vi "FTW-CodeGen-GetHelp.vi"(0 "State In":T4 {"Cache"."TotalCodeGens" format="CodeGens:   %04d"; "Cache"."TotalAdaptToInputs" format="AdaptTerms: %04d"; "Cache"."FinishedCodegen" format="%_3psec"; "Cache"."ElapsedTilCodegen" format="%_3psec"; "Cache"."AdaptToInputsBegin" format="%.3fmsec\n%<%D:%H:%M:%S%3u>t"}, 5 "XRef":refnum<vi>, 7 "Point":cluster{"Horizontal":i32, "Vertical":i32}) -> (4 "Standard Help Info":T3, 6 "Detailed Help Info":T2, 8 "Subitem Help Info":T1, 10 "Use Detailed Help?":bool, 15 "Use Subitem Help?":bool)   [LabVIEW 2015, in "FTW-SQLite-Insert.xnode"]
uses:
  FTW-CodeGen-State.ctl
  FTW-CodeGen-XNodeCommonState.ctl
  FTW-CodeGen-XNodeAdaptiveTerminal.ctl
  FTW-CodeGen-XNodeAdaptiveTerminal-Controller.ctl
  src/reflection/FTW-Reflection-Types.ctl
  FTW-CodeGen-XNodeAdaptiveTerminalWiringBehavior.ctl
  FTW-SQLite-Insert.xnode
panel:
  # "Inputs"
  # "Outputs"
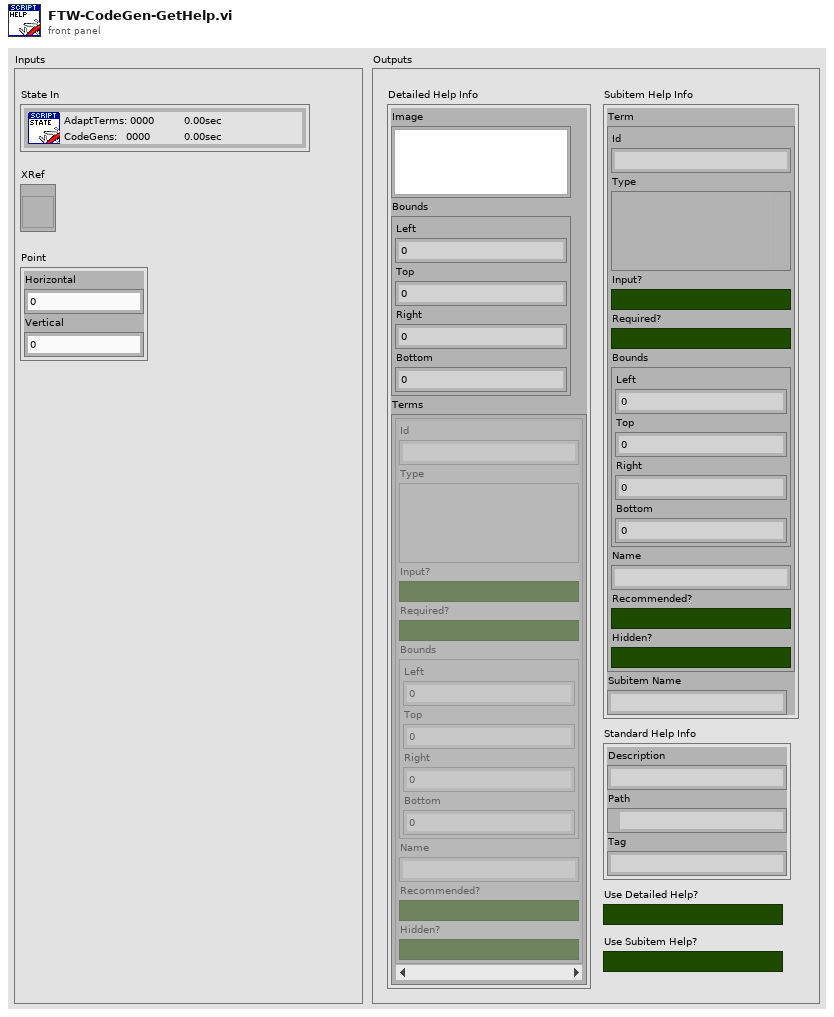
[diagram p1: front panel]
types:
  T1 = cluster{"Term":cluster{"Id":string, "Type":variant, "Input?":bool, "Required?":bool, "Bounds":cluster{"Left":i32, "Top":i32, "Right":i32, "Bottom":i32}, "Name":string, "Recommended?":bool, "Hidden?":bool}, "Subitem Name":string}
  T2 = cluster{"Image":picture, "Bounds":cluster{"Left":i32, "Top":i32, "Right":i32, "Bottom":i32}, "Terms":cluster{"Id":string, "Type":variant, "Input?":bool, "Required?":bool, "Bounds":cluster{"Left":i32, "Top":i32, "Right":i32, "Bottom":i32}, "Name":string, "Recommended?":bool, "Hidden?":bool}[]}
  T3 = cluster{"Description":string, "Path":path, "Tag":string}
  T4 = typedef "FTW-SQLite-Insert.xnode/FTW-CodeGen-State.ctl" = cluster{"Cache":T5}
  T5 = typedef "FTW-CodeGen-XNodeCommonState.ctl" = cluster{"Terms":cluster{"Name":string, "Id":string, "Type":variant, "Bounds":cluster{"Left":i32, "Top":i32, "Right":i32, "Bottom":i32}, "Input?":bool, "Required?":bool, "Recommended?":bool, "Adaptive?":bool, "Hidden?":bool, "Direction":enum32{"Auto", "Up", "Down", "Left", "Right", "Center"}, "Break Wire?":bool, "English Name":string}[], "AdaptiveTerms":T6[], "AdaptiveTerminalsOK":bool, "ForceCodeRegeneration?":bool, "LastGeneration":timestamp, "CodeGenError":errorcluster, "AdaptToInputsBegin":dbl, "ElapsedTilCodegen":dbl, "FinishedCodegen":dbl, "TotalAdaptToInputs":i32, "TotalCodeGens":i32}
  T6 = typedef "FTW-CodeGen-XNodeAdaptiveTerminal.ctl" = cluster{"Config":T7, "ID":string, "ParentIndex":i32, "Wired?":bool, "WiredTypeAllowed?":bool, "LastValidWireName":string, "LastValidWireType":T8, "Followers":i32[]}
  T7 = typedef "FTW-CodeGen-XNodeAdaptiveTerminal-Controller.ctl" = cluster{"AllowedTypes":T8[], "UnconstrainedTypeBehavior":T9, "DefaultType":variant}
  T8 = typedef "FTW-Reflection-Types.ctl" = enum16{"Unknown", "Void", "Array", "Cluster", "LVObject", "Boolean", "I8", "I16", "I32", "I64", "U8", "U16", "U32", "U64", "SGL", "DBL", "EXT", "CSG", "CDB", "CXT", "FXP", "EnumU8", "EnumU16", "EnumU32", "EnumU64", "SGLwithUnit", "DBLwithUnit", "EXTwithUnit", "CSGwithUnit", "CDBwithUnit", "CXTwithUnit", "String", "Path", "Picture", "Tag", "LVVariant", "Timestamp", "WaveformI8", "WaveformI16", "WaveformI32", "WaveformI64", "WaveformU8", "WaveformU16", "WaveformU32", "WaveformU64", "WaveformSGL", "WaveformDBL", "WaveformEXT", "WaveformCSG", "WaveformCDB", "WaveformCXT", "WaveformDigital", "WaveformUnknownType", "DigitalData", "DynamicData", "ExternalData", "FileByteStream", "TDMStream", "dotNET", "ActiveX", "VIServerReference", "VIReference", "ApplicationInstance", "Menu", "ConnectionDataSocket", "ConnectionVISA", "ConnectionBluetooth", "ConnectionIrDA", "ConnectionTCP", "ConnectionUDP", "ConnectionHTTPClient", "ConnectionFTP", "Occurrence", "Notifier", "Queue", "Rendezvous", "Semaphore", "RTFIFO", "EventPublisher", "EventRegistration", "EventCallback", "DataValueReference", "GenericClass", "GenericClassTag", "GenericClassDeepCopy", "GenericClassFlattened", "GenericClassTagFlattened", "GenericReferenceType", "WindowsRegistry", "OverloadedDatalogRef", "ReferenceUnknownType", "ByteArray", "ConPaneInterface", "FTWObject"}
  T9 = typedef "FTW-CodeGen-XNodeAdaptiveTerminalWiringBehavior.ctl" = enum16{"UseDefaultType", "StickyToLastValidType"}
  T10 = cluster{"Id":string, "Type":variant, "Input?":bool, "Required?":bool, "Bounds":cluster{"Left":i32, "Top":i32, "Right":i32, "Bottom":i32}, "Name":string, "Recommended?":bool, "Hidden?":bool}
  T11 = cluster{"Name":string, "Id":string, "Type":variant, "Bounds":cluster{"Left":i32, "Top":i32, "Right":i32, "Bottom":i32}, "Input?":bool, "Required?":bool, "Recommended?":bool, "Adaptive?":bool, "Hidden?":bool, "Direction":enum32{"Auto", "Up", "Down", "Left", "Right", "Center"}, "Break Wire?":bool, "English Name":string}[]
  T12 = cluster{"Left":i32, "Top":i32, "Right":i32, "Bottom":i32}
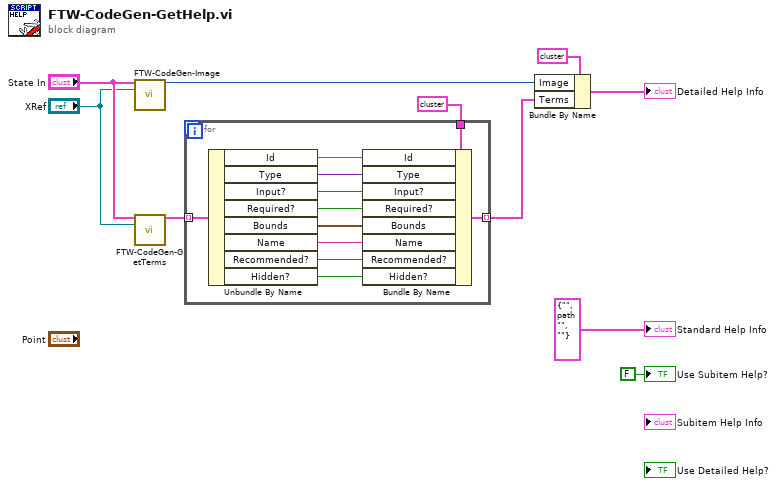
[diagram p0: block diagram]
diagram:
  n1 = call "FTW-CodeGen-Image.vi"("State In"="State In", "XRef"="XRef") -> ("Image"=w7:picture)  [unwired: 13 in]
  n2 = call "FTW-CodeGen-GetTerms.vi"("State In"="State In", "XRef"="XRef") -> ("Terms"=w4:T11)  [unwired: 13 in]
  n3 = for {
    tunnel: [w20] -> w6 mode=indexing
    tunnel: T10 {"Id"="", "Type"=variant, "Input?"=FALSE, "Required?"=FALSE, "Bounds"={"Left"=0, "Top"=0, "Right"=0, "Bottom"=0}, "Name"="", "Recommended?"=FALSE, "Hidden?"=FALSE} ("Term") -> [w21]
    tunnel: w4 -> [w19] mode=indexing
    n4 = Unbundle By Name(w19) -> ("Id"=w18:string, "Type"=w17:variant, "Input?"=w16:bool, "Required?"=w15:bool, "Bounds"=w14:T12, "Name"=w13:string, "Recommended?"=w12:bool, "Hidden?"=w11:bool)
    n5 = Bundle By Name(cluster=w21, "Id"=w18, "Type"=w17, "Input?"=w16, "Required?"=w15, "Bounds"=w14, "Name"=w13, "Recommended?"=w12, "Hidden?"=w11) -> (w20:T10)
  }
  n6 = Bundle By Name(cluster=T2 {"Image"=bytes[0], "Bounds"={"Left"=0, "Top"=0, "Right"=0, "Bottom"=0}, "Terms"=[]} ("Detailed Help Info"), "Image"=w7, "Terms"=w6) -> (→"Detailed Help Info":T2)
  "Standard Help Info" <- T3 {"Description"="", "Path"=path "", "Tag"=""} ("Standard Help Info")
  "Use Subitem Help?" <- FALSE ("Use Subitem Help?")
